vi "Re-order Protection Configs.vi"(11 "Protection Configurations":T1[](array[typedef]) {"CRC Channels"."Data Type" items=["Signed", "Unsigned", "IEEE Float"]}) -> (3 "Protection Configurations Out":T1[](array[typedef]) {"CRC Channels"."Data Type" items=["Signed", "Unsigned", "IEEE Float"]})   [LabVIEW 2023, in "LP_CRC.lvlib"]
uses:
  LP_CRC.lvlib
  Shared/Types/Exported Protection Settings.ctl
  Shared/Types/Protection Type.ctl
  Shared/Types/XNET Signal Configuration.ctl
  Shared/Protection and Counter Support Shared.lvlib
  <vilib>/Utility/SystemLogging/NI_SystemLogging.lvlib
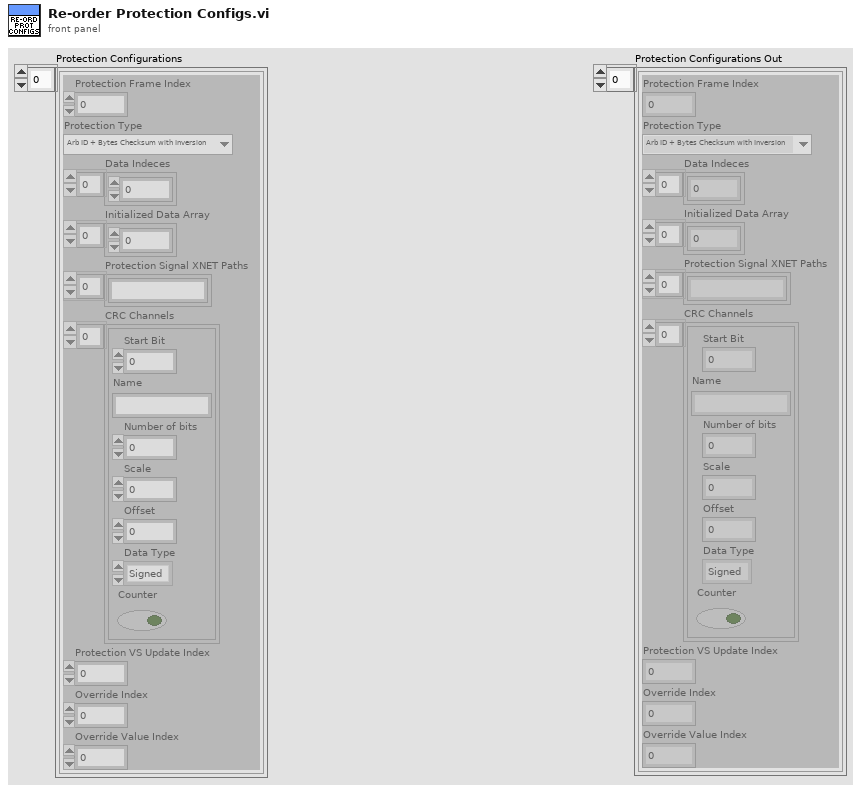
[diagram p1: front panel]
types:
  T1 = typedef "Protection and Counter Support Shared.lvlib/Exported Protection Settings.ctl" = cluster{"Protection Frame Index":i32, "Protection Type":T2, "Data Indeces":i32[], "Initialized Data Array":dbl[], "Protection Signal XNET Paths":string[], "CRC Channels":T3[], "Protection VS Update Index":i32, "Override Index":i32, "Override Value Index":i32}
  T2 = typedef "Protection and Counter Support Shared.lvlib/Protection Type.ctl" = enum16{"Arb ID + Bytes Checksum with Inversion", "Arb ID + Bytes CRC with Inversion", "Reversed Raw Signal Checksum with Inversion", "Concatenated Two's Compliment", "LP_CRC8", "LP_Checksum", "LP_CRC8_MRS"}
  T3 = typedef "Protection and Counter Support Shared.lvlib/XNET Signal Configuration.ctl" = cluster{"Start Bit":i32, "Name":string, "Number of bits":i32, "Scale":dbl, "Offset":dbl, "Data Type":u32, "Counter":bool}
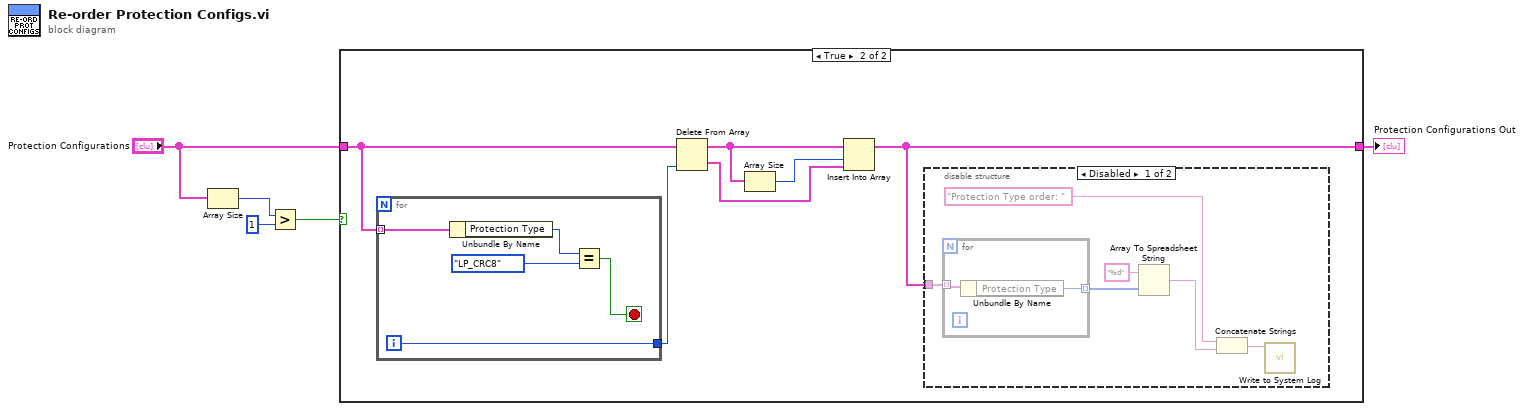
[diagram p0: block diagram]
diagram:
  n1 = Array Size(array="Protection Configurations") -> (size(s)=w4:i32)
  n2 = Greater?(x=w4, y=1) -> (0:w2:bool)
  n3 = case shown="True" w2 {
    tunnel: "Protection Configurations" -> [w6 w12]
    tunnel: [w6 w7] -> w1
    frame False {
    }
    frame True {
      n4 = for {
        tunnel: w12 -> [w25] mode=indexing
        tunnel: [w21] -> w11
        i -> [w21]
        stop <- w22 stop-if-true
        n5 = Unbundle By Name(w25) -> ("Protection Type"=w24:T2)
        n6 = Equal?(x=w24, y=Protection_Type."LP_CRC8") -> (x = y?=w22:bool)
      }
      n7 = Delete From Array "Delete From Array"(array=w12, index=w11) -> (deleted portion=w8:T1, array with subset deleted=w10:T1[])  [unwired: 1 in]
      n8 = Array Size(array=w10) -> (size(s)=w9:i32)
      n9 = Insert Into Array "Insert Into Array"(array=w10, index=w9, new element=w8) -> (w7:T1[])
      n10 = disable-structure shown="Disabled" {
        disable-tunnel: w7 -> [w18 _]
        frame Disabled {
          n11 = for {
            tunnel: w18 -> [w20] mode=indexing
            tunnel: [w19] -> w15 mode=indexing
            n12 = Unbundle By Name(w20) -> ("Protection Type"=w19:T2)
          }
          n13 = Array To Spreadsheet String(array=w15, 3:"%d" ("format string")) -> (spreadsheet string=w16:string)  [unwired: 1 in]
          n14 = Concatenate Strings("Protection Type order: " ("string"), w16) -> (w17:string)
          n15 = call <vilib>:"Write to System Log.vi"("message"=w17) -> ()  [unwired: 10 in, 1 out]
        }
        frame Enabled {
        }
      }
    }
  }
  "Protection Configurations Out" <- w1
